vi "Poly_One_Button.vi"(8 "error in":errorcluster, 10 "Button Text":string, 11 "Message":string) -> (0 "error out":errorcluster, 3 "Indicator 1":bool)   [LabVIEW 2024, in "Launcher_DTU.lvlib"]
uses:
  Launcher_DTU.lvlib
panel:
  out "Message":string
  in  "Button 1":bool
  # "Attention !"
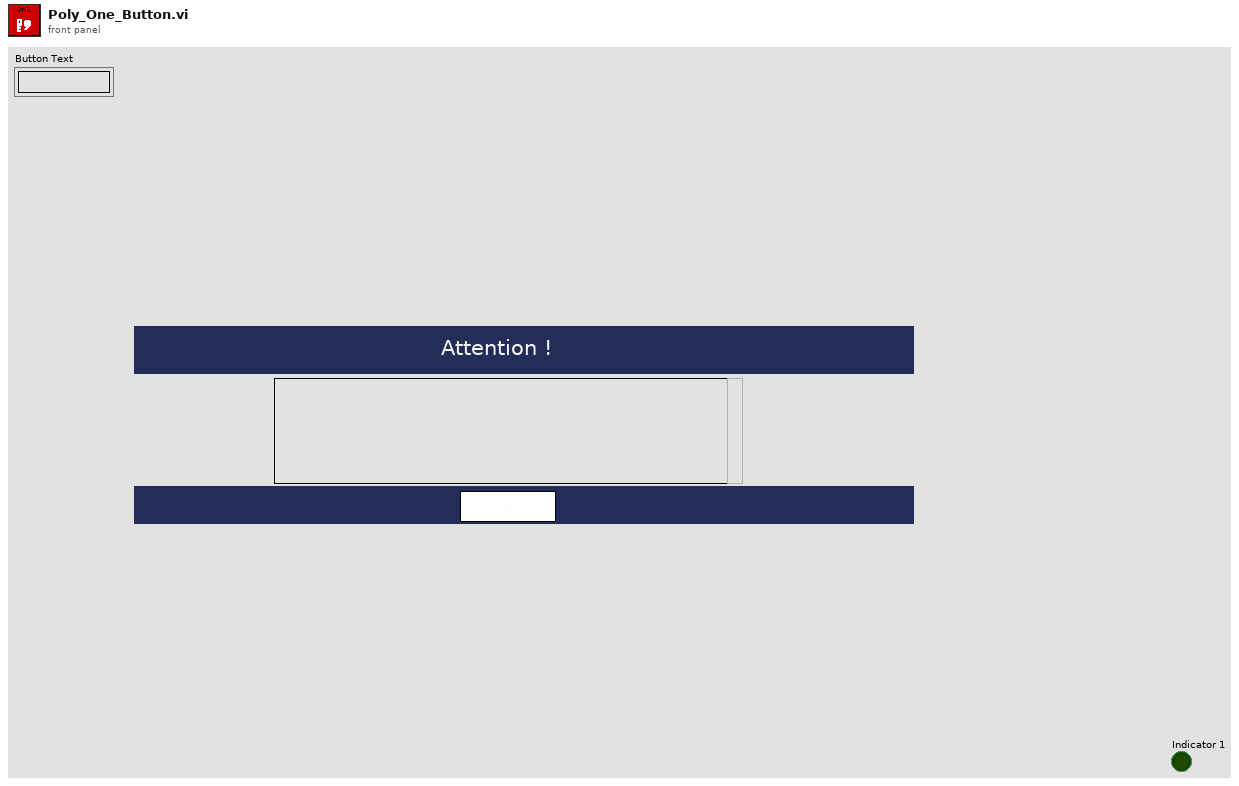
[diagram p1: front panel]
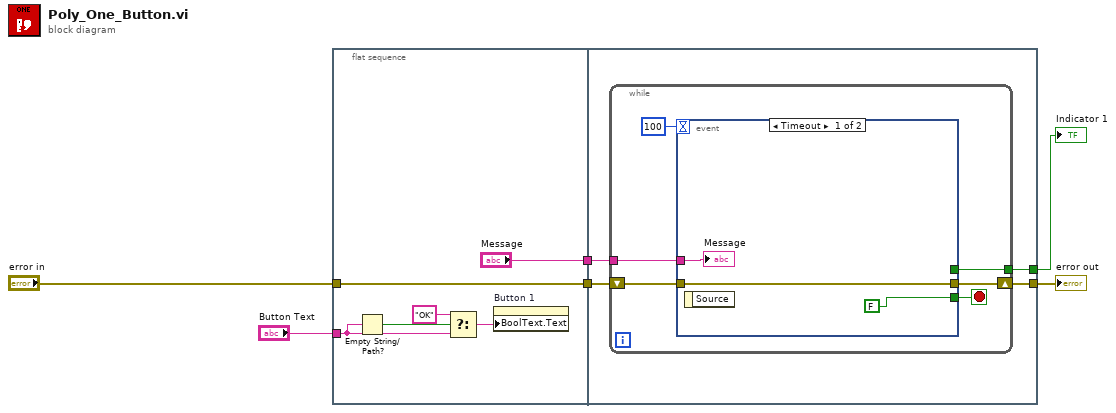
[diagram p0: block diagram]
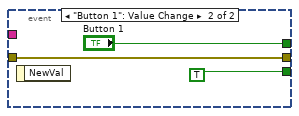
[diagram p2: hidden frame]
diagram:
  n1 = flat-sequence {
    tunnel: [w12] -> w5
    tunnel: "error in" -> [w12]
    tunnel: "Button Text" -> [w10]
    tunnel: ["Message"] -> w1
    tunnel: [w16] -> w6
    tunnel: w5 -> [w15]
    tunnel: [w14] -> w2
    tunnel: w1 -> [w13]
    frame #0 {
      n2 = Empty String/Path?(string/path=w10) -> (empty?=w11:bool)
      n3 = Select(t="OK", s=w11, f=w10) -> (s? t:f=w9:string)
      n4 = property on="Button 1" class="Bool"("BoolText.Text"=w9) -> ()  [unwired: 2 in, 2 out]
    }
    frame #1 {
      n5 = while {
        shift-right: [w20] -> w16
        shift-left: w15 -> [w21]
        tunnel: [w19] -> w14
        tunnel: w13 -> [w17]
        stop <- w18 stop-if-true
        n6 = event shown="[0] Timeout" {
          selector: _ -> [_ _]
          dyn-events: _ -> [_ _]
          timeout: 100 -> [_ _]
          tunnel: [FALSE TRUE] -> w18
          tunnel: w21 -> [w23 w27]
          tunnel: [w23 w27] -> w20
          tunnel: [_ "Button 1"] -> w19
          tunnel: w17 -> [w25 _]
          event Timeout {
            n7 = event-data() -> ()  [unwired: 1 in, 1 out]
            "Message" <- w25
          }
          event "Button 1": Value Change {
            n8 = event-data() -> ()  [unwired: 1 in, 1 out]
          }
        }
      }
    }
  }
  "error out" <- w6
  "Indicator 1" <- w2
